vi "Register Dynamic Events.vi"(8 "error in (no error)":errorcluster, 11 "TreeControlEventHandler In":refnum<class "TreeControlEventHandler.lvclass">) -> (0 "error out":errorcluster, 3 "TreeControlEventHandler Out":refnum<class "TreeControlEventHandler.lvclass">)   [LabVIEW 2015, in "ActorEvents.lvlib" / "TreeControlEventHandler.lvclass"]
uses:
  TreeControlEventHandler.lvclass
  IEventHandler/IEventHandler.lvclass/IEventHandler.ctl
  <vilib>/event_ctls.llb/lveventtype.ctl
  TreeControlEventHandler.lvclass/TreeControlEventHandler.ctl
  IEventHandler/Read Registrations.vi
  IEventHandler/IEventHandler.lvclass
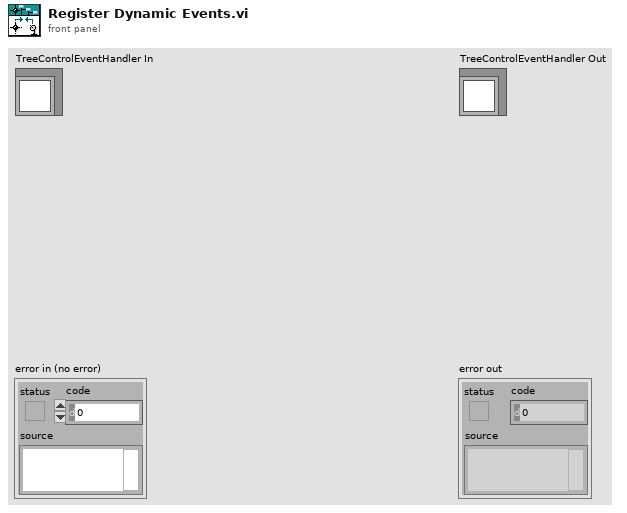
[diagram p1: front panel]
types:
  T1 = typedef "lveventtype.ctl" = enum32{"Null", "Timeout", "Annotation Menu Selection", "Annotation Menu Selection?", "App Instance Close", "App Instance Close?", "Autoscale Range Change", "Bookmark Info Change", "Cell Edit", "Cell Edit?", "Cursor Grab", "Cursor Grab?", "Cursor Menu Selection", "Cursor Menu Selection?", "Cursor Move", "Cursor Release", "Data Change", "Direction Change", "Display State Change", "Drag Ended", "Drag Enter", "Drag Leave", "Drag Over", "Drag Source Update", "Drag Starting", "Drag Starting?", "Drop", "Exec State Change", "Key Down", "Key Down?", "Key Repeat", "Key Repeat?", "Key Up", "Listbox Double Click", "Menu Activation?", "Menu Selection (App)", "Menu Selection? (App)", "Menu Selection (User)", "Mouse Down", "Mouse Down?", "Mouse Enter", "Mouse Leave", "Mouse Move", "Mouse Up", "Mouse Wheel", "NI Security User Change (App)", "Pane Size", "Panel Close", "Panel Close?", "Panel Resize", "Plot Attribute Change", "Scale Range Change", "Shortcut Menu Activation?", "Shortcut Menu Selection (App)", "Shortcut Menu Selection? (App)", "Shortcut Menu Selection (User)", "Tree Double Click", "Tree Drag", "Tree Drag?", "Tree Drop", "Tree Drop?", "Tree Item Close", "Tree Item Close?", "Tree Item Open", "Tree Item Open?", "User Event", "Value Change"}
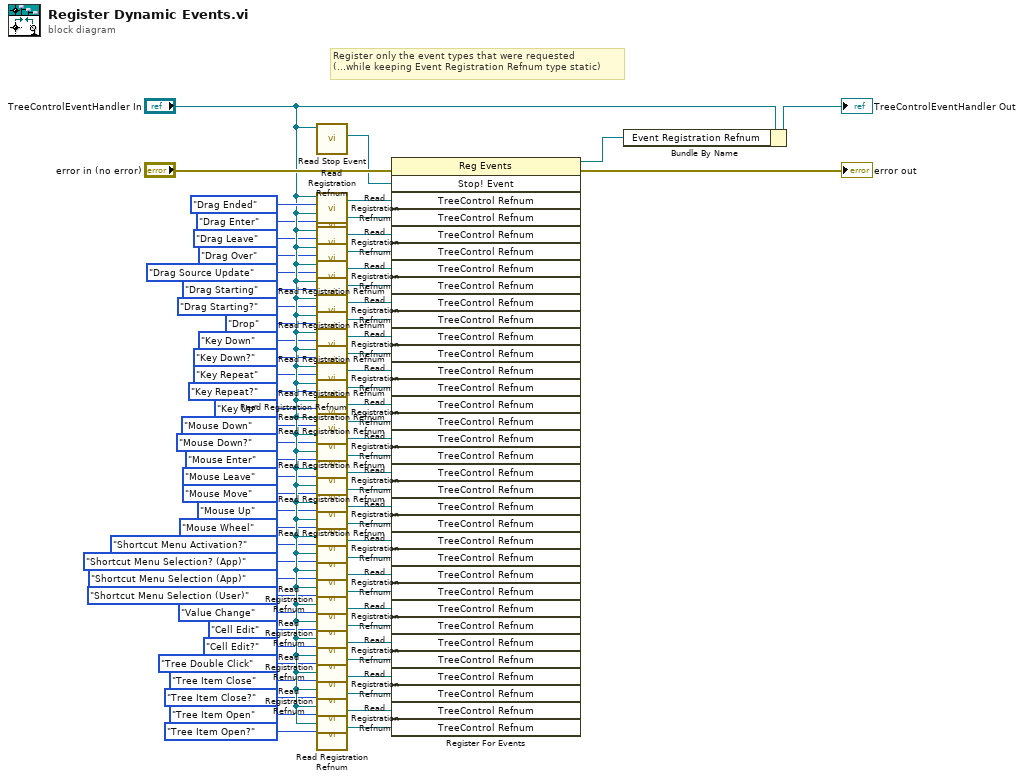
[diagram p0: block diagram]
diagram:
  # "Register only the event types that were requested\n(...while keeping Event Registration Refnum type static)"
  n1 = call "Read Stop Event.vi"("IEventHandler in"="TreeControlEventHandler In") -> ("Stop! Event"=w69:refnum<user-event>)  [unwired: 10 in]
  n2 = call "Read Registration Refnum.vi"("Event Type"=lveventtype."Drag Ended", "TreeControlEventHandler"="TreeControlEventHandler In") -> ("TreeControl Refnum"=w65:refnum<vi>)  [unwired: 5 in]
  n3 = call "Read Registration Refnum.vi"("Event Type"=lveventtype."Drag Enter", "TreeControlEventHandler"="TreeControlEventHandler In") -> ("TreeControl Refnum"=w63:refnum<vi>)  [unwired: 5 in]
  n4 = call "Read Registration Refnum.vi"("Event Type"=lveventtype."Drag Leave", "TreeControlEventHandler"="TreeControlEventHandler In") -> ("TreeControl Refnum"=w62:refnum<vi>)  [unwired: 5 in]
  n5 = call "Read Registration Refnum.vi"("Event Type"=lveventtype."Drag Over", "TreeControlEventHandler"="TreeControlEventHandler In") -> ("TreeControl Refnum"=w61:refnum<vi>)  [unwired: 5 in]
  n6 = call "Read Registration Refnum.vi"("Event Type"=lveventtype."Drag Source Update", "TreeControlEventHandler"="TreeControlEventHandler In") -> ("TreeControl Refnum"=w60:refnum<vi>)  [unwired: 5 in]
  n7 = call "Read Registration Refnum.vi"("Event Type"=lveventtype."Drag Starting", "TreeControlEventHandler"="TreeControlEventHandler In") -> ("TreeControl Refnum"=w59:refnum<vi>)  [unwired: 5 in]
  n8 = call "Read Registration Refnum.vi"("Event Type"=lveventtype."Drag Starting?", "TreeControlEventHandler"="TreeControlEventHandler In") -> ("TreeControl Refnum"=w58:refnum<vi>)  [unwired: 5 in]
  n9 = call "Read Registration Refnum.vi"("Event Type"=lveventtype."Drop", "TreeControlEventHandler"="TreeControlEventHandler In") -> ("TreeControl Refnum"=w57:refnum<vi>)  [unwired: 5 in]
  n10 = call "Read Registration Refnum.vi"("Event Type"=lveventtype."Key Down", "TreeControlEventHandler"="TreeControlEventHandler In") -> ("TreeControl Refnum"=w56:refnum<vi>)  [unwired: 5 in]
  n11 = call "Read Registration Refnum.vi"("Event Type"=lveventtype."Key Down?", "TreeControlEventHandler"="TreeControlEventHandler In") -> ("TreeControl Refnum"=w55:refnum<vi>)  [unwired: 5 in]
  n12 = call "Read Registration Refnum.vi"("Event Type"=lveventtype."Key Repeat", "TreeControlEventHandler"="TreeControlEventHandler In") -> ("TreeControl Refnum"=w54:refnum<vi>)  [unwired: 5 in]
  n13 = call "Read Registration Refnum.vi"("Event Type"=lveventtype."Key Repeat?", "TreeControlEventHandler"="TreeControlEventHandler In") -> ("TreeControl Refnum"=w53:refnum<vi>)  [unwired: 5 in]
  n14 = call "Read Registration Refnum.vi"("Event Type"=lveventtype."Key Up", "TreeControlEventHandler"="TreeControlEventHandler In") -> ("TreeControl Refnum"=w52:refnum<vi>)  [unwired: 5 in]
  n15 = call "Read Registration Refnum.vi"("Event Type"=lveventtype."Mouse Down", "TreeControlEventHandler"="TreeControlEventHandler In") -> ("TreeControl Refnum"=w51:refnum<vi>)  [unwired: 5 in]
  n16 = call "Read Registration Refnum.vi"("Event Type"=lveventtype."Mouse Down?", "TreeControlEventHandler"="TreeControlEventHandler In") -> ("TreeControl Refnum"=w50:refnum<vi>)  [unwired: 5 in]
  n17 = call "Read Registration Refnum.vi"("Event Type"=lveventtype."Mouse Enter", "TreeControlEventHandler"="TreeControlEventHandler In") -> ("TreeControl Refnum"=w49:refnum<vi>)  [unwired: 5 in]
  n18 = call "Read Registration Refnum.vi"("Event Type"=lveventtype."Mouse Leave", "TreeControlEventHandler"="TreeControlEventHandler In") -> ("TreeControl Refnum"=w48:refnum<vi>)  [unwired: 5 in]
  n19 = call "Read Registration Refnum.vi"("Event Type"=lveventtype."Mouse Move", "TreeControlEventHandler"="TreeControlEventHandler In") -> ("TreeControl Refnum"=w47:refnum<vi>)  [unwired: 5 in]
  n20 = call "Read Registration Refnum.vi"("Event Type"=lveventtype."Mouse Up", "TreeControlEventHandler"="TreeControlEventHandler In") -> ("TreeControl Refnum"=w46:refnum<vi>)  [unwired: 5 in]
  n21 = call "Read Registration Refnum.vi"("Event Type"=lveventtype."Mouse Wheel", "TreeControlEventHandler"="TreeControlEventHandler In") -> ("TreeControl Refnum"=w45:refnum<vi>)  [unwired: 5 in]
  n22 = call "Read Registration Refnum.vi"("Event Type"=lveventtype."Shortcut Menu Activation?", "TreeControlEventHandler"="TreeControlEventHandler In") -> ("TreeControl Refnum"=w44:refnum<vi>)  [unwired: 5 in]
  n23 = call "Read Registration Refnum.vi"("Event Type"=lveventtype."Shortcut Menu Selection? (App)", "TreeControlEventHandler"="TreeControlEventHandler In") -> ("TreeControl Refnum"=w43:refnum<vi>)  [unwired: 5 in]
  n24 = call "Read Registration Refnum.vi"("Event Type"=lveventtype."Shortcut Menu Selection (App)", "TreeControlEventHandler"="TreeControlEventHandler In") -> ("TreeControl Refnum"=w42:refnum<vi>)  [unwired: 5 in]
  n25 = call "Read Registration Refnum.vi"("Event Type"=lveventtype."Shortcut Menu Selection (User)", "TreeControlEventHandler"="TreeControlEventHandler In") -> ("TreeControl Refnum"=w41:refnum<vi>)  [unwired: 5 in]
  n26 = call "Read Registration Refnum.vi"("Event Type"=lveventtype."Value Change", "TreeControlEventHandler"="TreeControlEventHandler In") -> ("TreeControl Refnum"=w40:refnum<vi>)  [unwired: 5 in]
  n27 = call "Read Registration Refnum.vi"("Event Type"=lveventtype."Cell Edit", "TreeControlEventHandler"="TreeControlEventHandler In") -> ("TreeControl Refnum"=w39:refnum<vi>)  [unwired: 5 in]
  n28 = call "Read Registration Refnum.vi"("Event Type"=lveventtype."Cell Edit?", "TreeControlEventHandler"="TreeControlEventHandler In") -> ("TreeControl Refnum"=w38:refnum<vi>)  [unwired: 5 in]
  n29 = call "Read Registration Refnum.vi"("Event Type"=lveventtype."Tree Double Click", "TreeControlEventHandler"="TreeControlEventHandler In") -> ("TreeControl Refnum"=w37:refnum<vi>)  [unwired: 5 in]
  n30 = call "Read Registration Refnum.vi"("Event Type"=lveventtype."Tree Item Close", "TreeControlEventHandler"="TreeControlEventHandler In") -> ("TreeControl Refnum"=w36:refnum<vi>)  [unwired: 5 in]
  n31 = call "Read Registration Refnum.vi"("Event Type"=lveventtype."Tree Item Close?", "TreeControlEventHandler"="TreeControlEventHandler In") -> ("TreeControl Refnum"=w35:refnum<vi>)  [unwired: 5 in]
  n32 = call "Read Registration Refnum.vi"("Event Type"=lveventtype."Tree Item Open", "TreeControlEventHandler"="TreeControlEventHandler In") -> ("TreeControl Refnum"=w34:refnum<vi>)  [unwired: 5 in]
  n33 = call "Read Registration Refnum.vi"("Event Type"=lveventtype."Tree Item Open?", "TreeControlEventHandler"="TreeControlEventHandler In") -> ("TreeControl Refnum"=w64:refnum<vi>)  [unwired: 5 in]
  n34 = register-events(error in="error in (no error)", w69, w65, w63, w62, w61, w60, w59, w58, w57, w56, w55, w54, w53, w52, w51, w50, w49, w48, w47, w46, w45, w44, w43, w42, w41, w40, w39, w38, w37, w36, w35, w34, w64) -> (reference out=w1:refnum<event-registration>, error out=→"error out":errorcluster)  [unwired: 1 in]
  n35 = Bundle By Name(cluster="TreeControlEventHandler In", "Event Registration Refnum"=w1) -> (→"TreeControlEventHandler Out":refnum<class "TreeControlEventHandler.lvclass">)
